vi "Count down U8.vi"(9 "load":bool=TRUE, 10 "decrement":bool=TRUE, 11 "count in":u8) -> (1 "terminal count":bool, 2 "count out":u8)   [LabVIEW 2020]
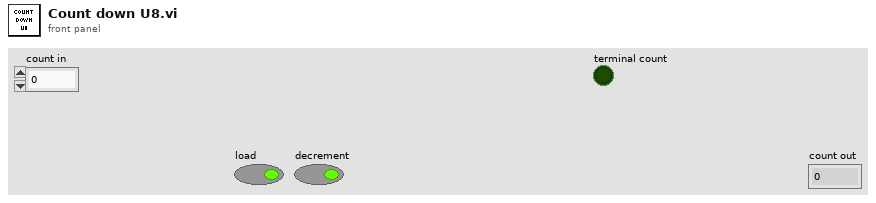
[diagram p1: front panel]
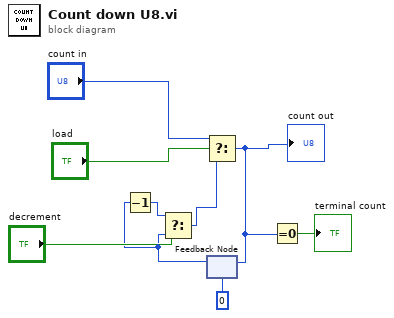
[diagram p0: block diagram]
diagram:
  n1 = feedback #1(u8 0) -> (w3:u8)
  n2 = Decrement(x=w3) -> (x-1=w4:u8)
  n3 = Select(t=w4, s="decrement", f=w3) -> (s? t:f=w6:u8)
  n4 = Select(t="count in", s="load", f=w6) -> (s? t:f=w2:u8)
  "count out" <- w2
  n5 = feedback-in #1(w2) -> ()
  n6 = Equal To 0?(x=w2) -> (x = 0?=→"terminal count":bool)
